vi "Post-Build Action.vi"(5 "Files Generated by Build":path[](array[path]), 6 "Top Level/Always Included VIs":path[](array[path]), 7 "Destination Path":path, 8 "error in (no error)":errorcluster, 9 "Target Name":string, 10 "Build Specification Name":string, 11 "Project Path":path) -> (0 "error out":errorcluster)   [LabVIEW 2015]
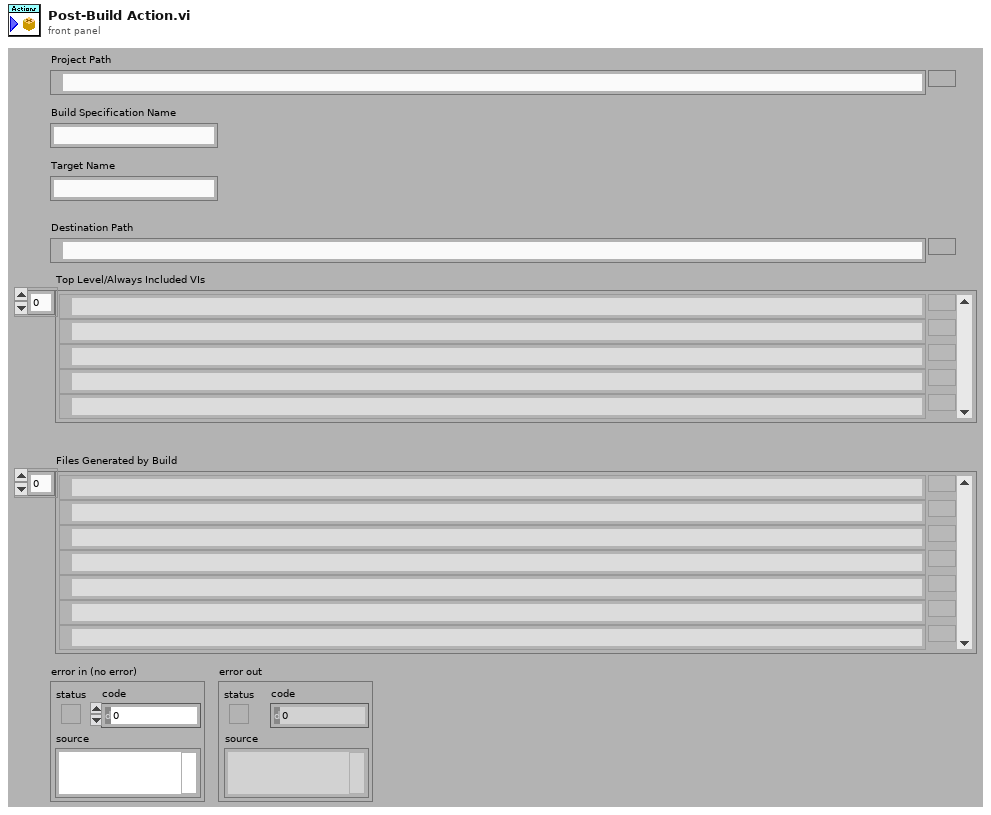
[diagram p1: front panel]
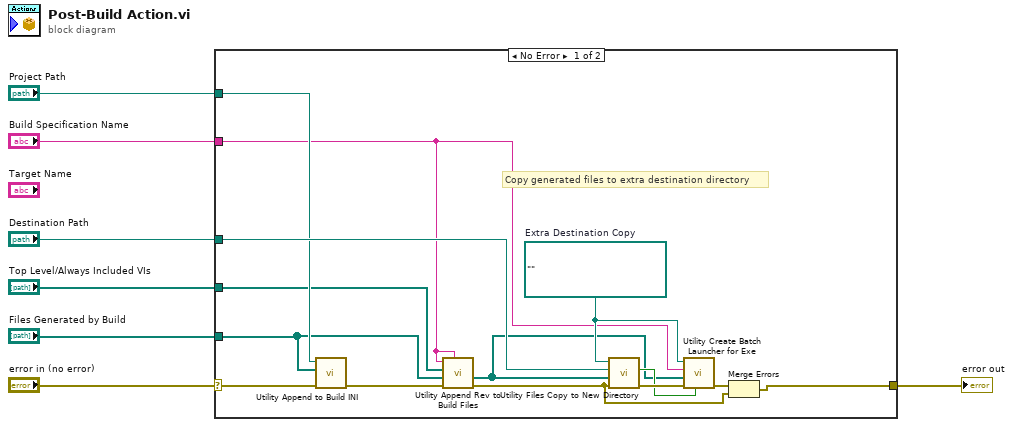
[diagram p0: block diagram]
diagram:
  n1 = case shown="No Error" "error in (no error)" {
    selector: "error in (no error)" -> [w19 w22]
    tunnel: "Files Generated by Build" -> [w10 _]
    tunnel: [w18 w22] -> w4
    tunnel: "Destination Path" -> [w21 _]
    tunnel: "Project Path" -> [w20 _]
    tunnel: "Build Specification Name" -> [w11 _]
    tunnel: "Top Level/Always Included VIs" -> [w8 _]
    frame No Error {
      w15 = path ""  # Extra Destination Copy
      # "Copy generated files to extra destination directory"
      n2 = call "Utility Append to Build INI.vi"("error in (no error)"=w19, "Files Generated by Build"=w10, "Project Path"=w20) -> ("error out"=w13:errorcluster)  [unwired: 8 in]
      n3 = call "Utility Append Rev to Build Files.vi"("Executable Name"=w11, "error in (no error)"=w13, "Files Generated by Build in"=w10, "Top Level/Always Included VIs"=w8, "Build Specification Name"=w11) -> ("error out"=w12:errorcluster, "Files Generated by Build out"=w9:path[])  [unwired: 5 in]
      n4 = call "Utility Files Copy to New Directory.vi"("error in (no error)"=w12, "All Files"=w9, "Base Folder"=w21, "New Base Folder"=w15) -> ("error out"=w17:errorcluster, "Copied?"=w14:bool)  [unwired: 6 in]
      n5 = call "Utility Create Batch Launcher for Exe.vi"("Enable (T)"=w14, "error in (no error)"=w17, "Files Generated by Build"=w9, "Build Specification Name"=w11, "Extra Destination Copy"=w15) -> ("error out"=w16:errorcluster)  [unwired: 6 in]
      n6 = Merge Errors(w16, w12) -> (w18:errorcluster)
    }
    frame Error {
    }
  }
  "error out" <- w4
